vi "ATF-Pump-AI C Start.vi"(8 "error in":errorcluster, 10 "AI C":T1(array[cluster]), 11 "Refnum in":refnum<k21>) -> (0 "error out":errorcluster, 3 "Refnum out":refnum<k21>)   [LabVIEW 2022 SP3]
uses:
  <vilib>/DAQmx/configure/timing.llb/DAQmx Timing (Sample Clock).vi
  <vilib>/DAQmx/configure/trigger.llb/DAQmx Start Trigger (Digital Edge).vi
  <resource>/objmgr/daqmx.rc
panel:
  in  "AI.DigFltr.Response 2":i32(ring)=10191 items=["Constant Group Delay"=16075, "Butterworth"=16076, "Elliptical"=16077, "Hardware Defined"=10191]
  in  "AI.DigFltr.Type 2":i32(ring)=16071 items=["Lowpass"=16071, "Highpass"=16072, "Bandpass"=16073, "Notch"=16074, "Custom"=10137]
  in  "AI.DigFltr.Lowpass.CutoffFreq 2":dbl=20.0
  in  "AI.DigFltr.Order 2":u32=4
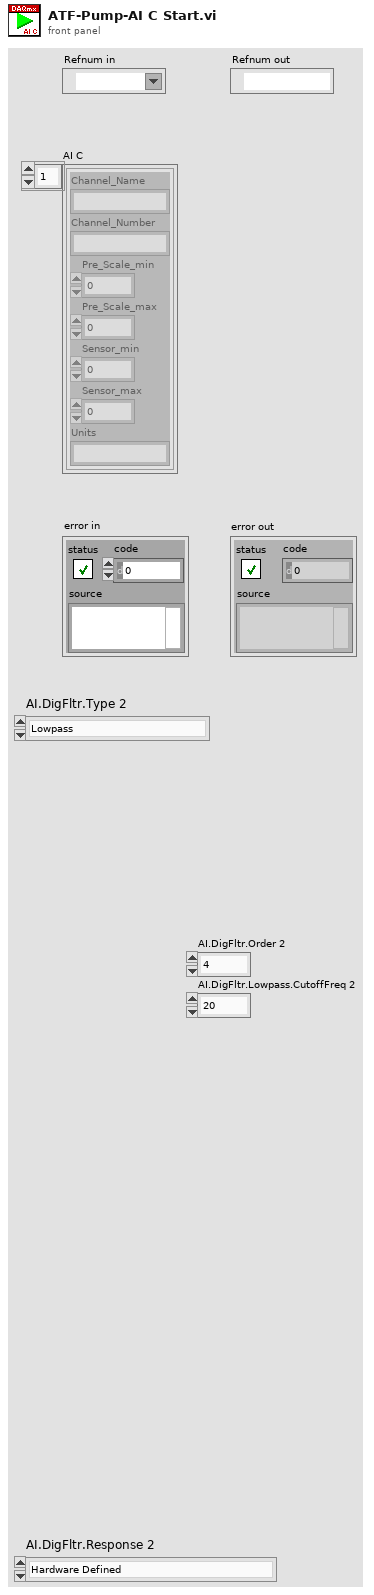
[diagram p1: front panel]
types:
  T1 = cluster{"Channel_Name":string, "Channel_Number":string, "Pre_Scale_min":dbl, "Pre_Scale_max":dbl, "Sensor_min":dbl, "Sensor_max":dbl, "Units":string}[]
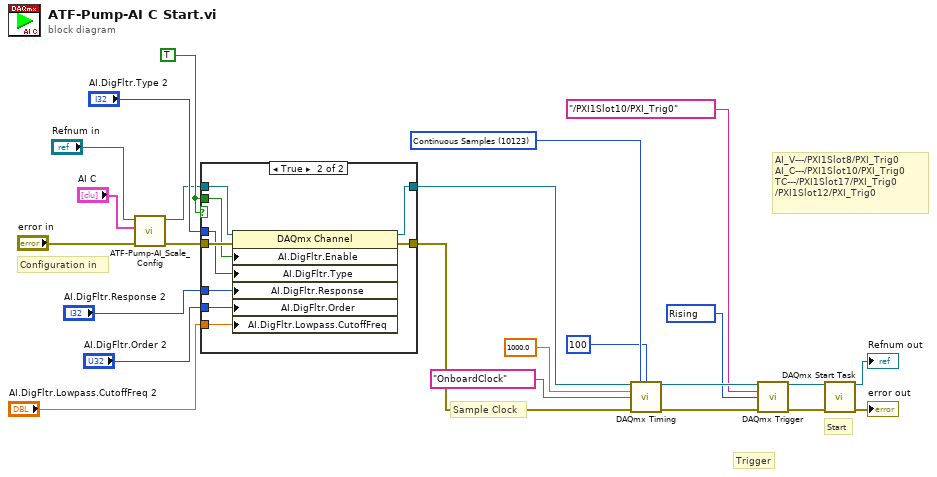
[diagram p0: block diagram]
diagram:
  w11 = TRUE
  w12 = 10280 items=["Rising"=10280, "Falling"=10171] ("edge")
  w20 = 10123 items=["Finite Samples"=10178, "Continuous Samples"=10123, "Hardware Timed Single Point"=12522] ("sample mode")
  # "AI_V---/PXI1Slot8/PXI_Trig0\nAI_C---/PXI1Slot10/PXI_Trig0\nTC---/PXI1Slot17/PXI_Trig0\n/PXI1Slot12/PXI_Trig0"
  # "Start"
  # "Trigger"
  # "Sample Clock"
  # "Configuration in"
  n1 = call "ATF-Pump-AI_Scale_Config.vi"("error in (no error)"="error in", "AI C"="AI C", "Refnum in"="Refnum in") -> ("error out"=w4:errorcluster, "Refnum out"=w6:refnum<k21>)  [unwired: 7 in]
  n2 = case shown="True" w11 {
    tunnel: w6 -> [w26 w35]
    tunnel: [w26 w34] -> w5
    tunnel: w4 -> [w25 w33]
    tunnel: [w25 w32] -> w3
    tunnel: w11 -> [_ w31]
    tunnel: "AI.DigFltr.Type 2" -> [_ w30]
    tunnel: "AI.DigFltr.Response 2" -> [_ w29]
    tunnel: "AI.DigFltr.Order 2" -> [_ w28]
    tunnel: "AI.DigFltr.Lowpass.CutoffFreq 2" -> [_ w27]
    frame False {
    }
    frame True {
      n3 = property class="DAQmx Channel"(reference=w35, error in=w33, "AI.DigFltr.Enable"=w31, "AI.DigFltr.Type"=w30, "AI.DigFltr.Response"=w29, "AI.DigFltr.Order"=w28, "AI.DigFltr.Lowpass.CutoffFreq"=w27) -> (reference out=w34:refnum<k21>, error out=w32:errorcluster)
    }
  }
  n4 = call-poly <vilib>:"DAQmx Timing.vi"("task/channels in"=w5, "sample mode"=w20, "samples per channel"=100, "rate"=1000.0, "source"=tag "OnboardClock", "error in"=w3) -> ("task out"=w23:refnum<k21>, "error out"=w14:errorcluster)  [unwired: 8 in]
  n5 = call-poly <vilib>:"DAQmx Trigger.vi"("task/channels in"=w23, "source"=tag "/PXI1Slot10/PXI_Trig0", "edge"=w12, "error in"=w14) -> ("task out"=w15:refnum<k21>, "error out"=w13:errorcluster)  [unwired: 10 in]
  n6 = call <vilib>:"DAQmx Start Task.vi"("task/channels in"=w15, "error in"=w13) -> ("task out"=→"Refnum out":refnum<k21>, "error out"=→"error out":errorcluster)  [unwired: 12 in]
